vi "BRig_Host_dataRunState_dataTS_sSelection.vi"() -> (2 "output_idx_dataTS_sSelection":i32)   [LabVIEW 2014]
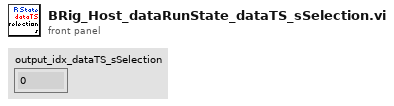
[diagram p1: front panel]
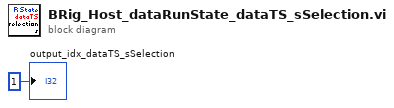
[diagram p0: block diagram]
diagram:
  "output_idx_dataTS_sSelection" <- 1 ("output_idx_dataTS")
